vi "Periodic Tasks.vi"(8 "error in":errorcluster) -> ()   [LabVIEW 2023]
doc: "This VI runs in parallel to other tasks. It can contain as many user-defined periodic loops as you need. These can carry out PID or other sorts of timed response."
uses:
  <vilib>/Rock Robotics/WPI/ThirdParty/REV Robotics/REVLib/Typedef/Spark MAX Smart Motion Parameters.ctl
  <vilib>/Rock Robotics/WPI/Utilities/WPI_GetSetVariantRefNum.vi
  <vilib>/Rock Robotics/WPI/RobotDrive/WPI_RobotDriveMecanumDrive_Cartesian.vi
panel:
  in  "Velocity PID Constants RB":T1={"P Gain"=0.0, "I Gain"=0.0, "D Gain"=0.0, "F Gain"=0.0, "I Zone"=0.0, "Min Output"=-1.0, "Max Output"=1.0} {"Max Output" min=-1.0 max=1.0 step=0.01; "Min Output" min=-1.0 max=1.0 step=0.01; "I Zone" step=0.01; "F Gain" step=0.01; "D Gain" step=0.01; "I Gain" step=0.01; "P Gain" min=0.0 step=0.01}
  in  "Smart Motion Parameters RB":T2={"Max Velocity"=2000.0, "Max Acceleration"=1500.0, "Minimum Velocity Output"=0.0, "Allowed Closed Loop Error"=0.0}
  in  "Velocity PID Constants LB":T1={"P Gain"=0.0, "I Gain"=0.0, "D Gain"=0.0, "F Gain"=0.0, "I Zone"=0.0, "Min Output"=-1.0, "Max Output"=1.0} {"Max Output" min=-1.0 max=1.0 step=0.01; "Min Output" min=-1.0 max=1.0 step=0.01; "I Zone" step=0.01; "F Gain" step=0.01; "D Gain" step=0.01; "I Gain" step=0.01; "P Gain" min=0.0 step=0.01}
  in  "Smart Motion Parameters LB":T2={"Max Velocity"=2000.0, "Max Acceleration"=1500.0, "Minimum Velocity Output"=0.0, "Allowed Closed Loop Error"=0.0}
  in  "Velocity PID Constants LF":T1={"P Gain"=0.0, "I Gain"=0.0, "D Gain"=0.0, "F Gain"=0.0, "I Zone"=0.0, "Min Output"=-1.0, "Max Output"=1.0} {"Max Output" min=-1.0 max=1.0 step=0.01; "Min Output" min=-1.0 max=1.0 step=0.01; "I Zone" step=0.01; "F Gain" step=0.01; "D Gain" step=0.01; "I Gain" step=0.01; "P Gain" min=0.0 step=0.01}
  in  "Smart Motion Parameters LF":T2={"Max Velocity"=2000.0, "Max Acceleration"=1500.0, "Minimum Velocity Output"=0.0, "Allowed Closed Loop Error"=0.0}
  in  "Velocity PID Constants RF":T1={"P Gain"=0.0, "I Gain"=0.0, "D Gain"=0.0, "F Gain"=0.0, "I Zone"=0.0, "Min Output"=-1.0, "Max Output"=1.0} {"Max Output" min=-1.0 max=1.0 step=0.01; "Min Output" min=-1.0 max=1.0 step=0.01; "I Zone" step=0.01; "F Gain" step=0.01; "D Gain" step=0.01; "I Gain" step=0.01; "P Gain" min=0.0 step=0.01}
  in  "Smart Motion Parameters RF":T2={"Max Velocity"=2000.0, "Max Acceleration"=1500.0, "Minimum Velocity Output"=0.0, "Allowed Closed Loop Error"=0.0}
  # "Click here to set max"
  # "Click here to set min"
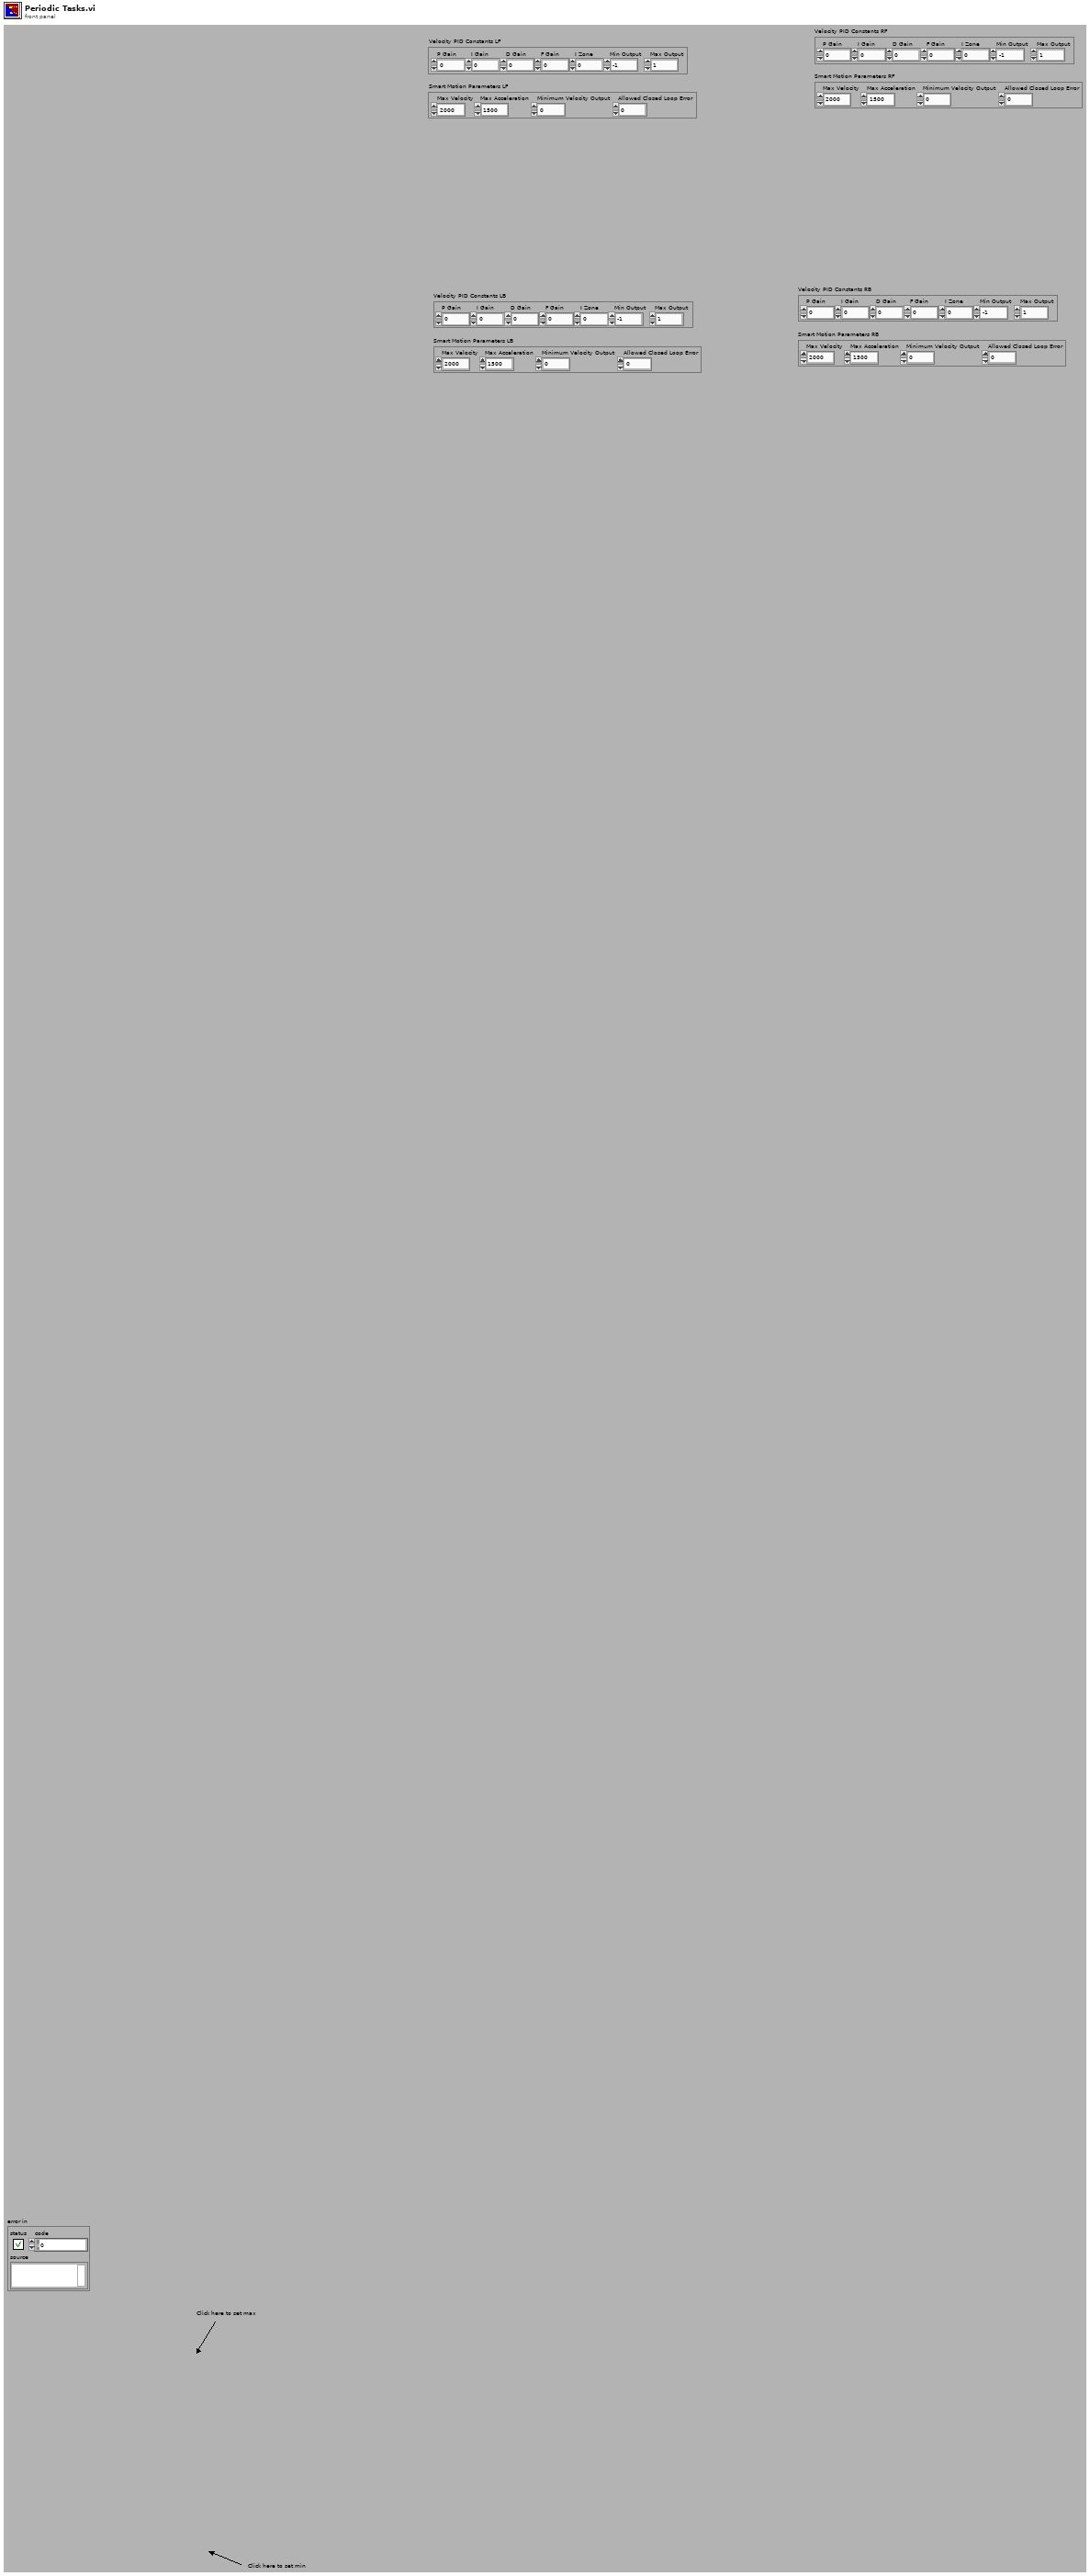
[diagram p1: front panel]
types:
  T1 = cluster{"P Gain":dbl, "I Gain":dbl, "D Gain":dbl, "F Gain":dbl, "I Zone":dbl, "Min Output":dbl, "Max Output":dbl}
  T2 = typedef "Spark MAX Smart Motion Parameters.ctl" = cluster{"Max Velocity":dbl, "Max Acceleration":dbl, "Minimum Velocity Output":dbl, "Allowed Closed Loop Error":dbl}
  T3 = typedef "WPI_JoystickDevRef.ctl" = cluster{"Device":T4}
  T4 = typedef "WPI_JoystickDeviceEnum.ctl" = enum16{"USB 0", "USB 1", "USB 2", "USB 3", "USB 4", "USB 5"}
  T5 = typedef "WPI_RobotDriveDevRef.ctl" = cluster{"DevStatus":errorcluster, "Motors[]":T6[], "Square Inputs":bool, "Max Output":dbl}
  T6 = typedef "WPI_MotorControlDeviceRef.ctl" = cluster{"DeviceStatus":errorcluster, "Type":T7, "PWM":cluster{"PWM Channel":T8, "DeadBand":T9}, "CAN":cluster{"Device Number":u8, "SetOutput VI Ref":variant, "GetOutput VI Ref":variant, "Enable VI Ref":variant, "Disable VI Ref":variant, "Data":variant}, "Invert":bool, "DIO PWM":cluster{"PWM \"Enable\" Channel":T8, "DIOChannel":T10, "PWM Rate":dbl}}
  T7 = typedef "WPI_MotorControlType.ctl" = enum16{"PWM", "CAN", "DIO PWM"}
  T8 = typedef "FPGA_DIOPWMChannel.ctl" = enum8{"PWM 0", "PWM 1", "PWM 2", "PWM 3", "PWM 4", "PWM 5", "PWM 6", "PWM 7", "PWM 8", "PWM 9", "PWM MXP 0", "PWM MXP 1", "PWM MXP 2", "PWM MXP 3", "PWM MXP 4", "PWM MXP 5", "PWM MXP 6", "PWM MXP 7", "PWM MXP 8", "PWM MXP 9", "Invalid"}
  T9 = typedef "WPI_PWMDeadband.ctl" = cluster{"Name":string, "maxPositivePwm":i32, "minPositivePwm":i32, "centerPwm":i32, "maxNegativePwm":i32, "minNegativePwm":i32, "angularRange":u16}
  T10 = typedef "FPGA_DIOChannel.ctl" = enum8{"DIO 0", "DIO 1", "DIO 2", "DIO 3", "DIO 4", "DIO 5", "DIO 6", "DIO 7", "DIO 8", "DIO 9", "DIO MXP 0", "DIO MXP 1", "DIO MXP 2", "DIO MXP 3", "DIO MXP 4", "DIO MXP 5", "DIO MXP 6", "DIO MXP 7", "DIO MXP 8", "DIO MXP 9", "DIO MXP 10", "DIO MXP 11", "DIO MXP 12", "DIO MXP 13", "DIO MXP 14", "DIO MXP 15", "SPI Port CS1", "SPI Port CS2", "SPI Port CS3", "SPI Port MISO", "SPI Port MOSI", "Invalid"}
  T11 = typedef "WPI_DigitalInputDevRef.ctl" = cluster{"DevStatus":errorcluster, "DIO Channel":T10}
  T12 = cluster{"JoystickDevRef":T3, "RobotDriveDevRef":T5}
  T13 = cluster{"P Gain":bool, "I Gain":bool, "D Gain":bool, "F Gain":bool, "I Zone":bool, "Min Output":bool, "Max Output":bool}
  T14 = cluster{"Max Velocity":bool, "Max Acceleration":bool, "Minimum Velocity Output":bool, "Allowed Closed Loop Error":bool}
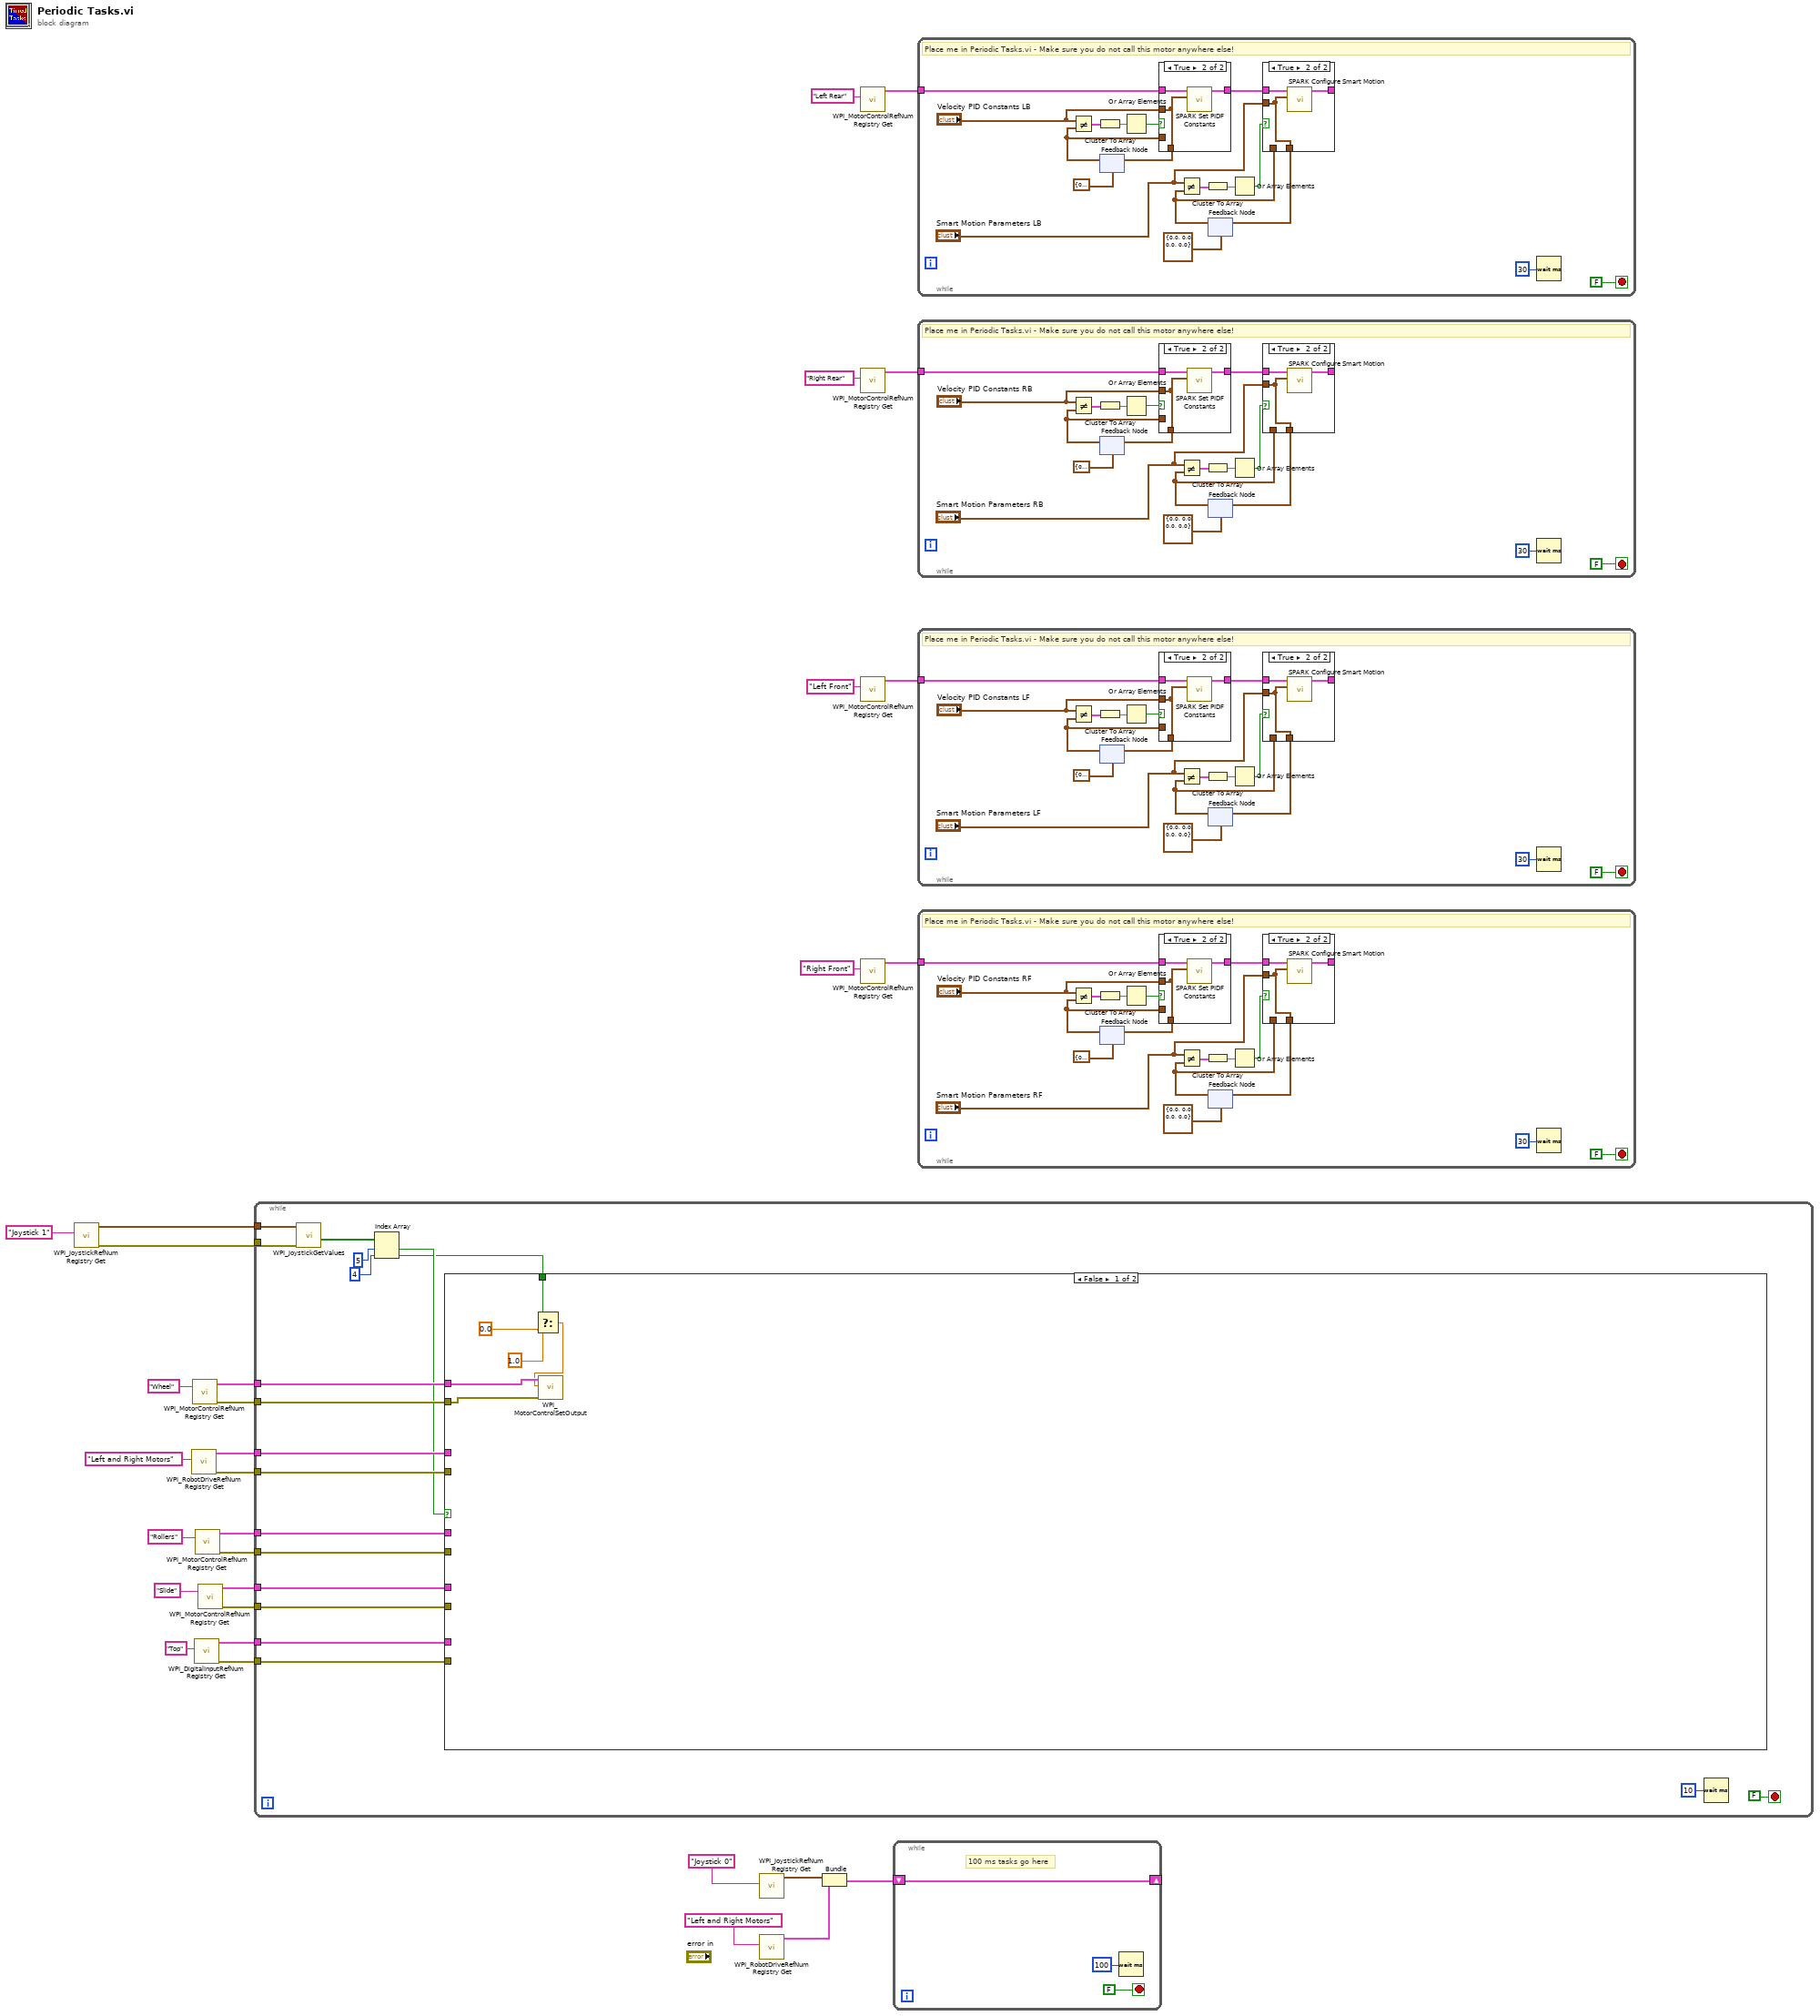
[diagram p0: block diagram]
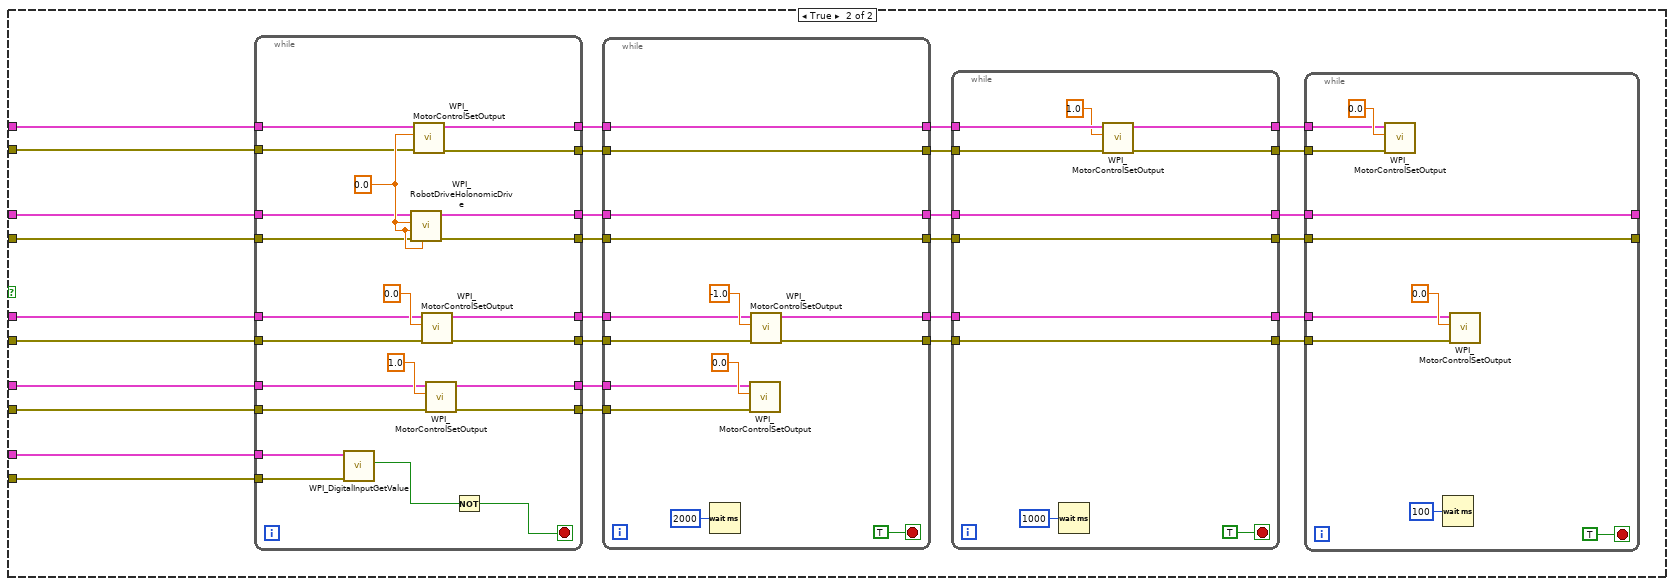
[diagram p10: hidden frame]
diagram:
  n1 = call <vilib>:"WPI_JoystickRefNum Registry Get.vi"("refnum name"="Joystick 1") -> ("error out"=w2:errorcluster, "JoystickDevRef"=w1:T3)  [unwired: 1 in, 8 out]
  n2 = call <vilib>:"WPI_RobotDriveRefNum Registry Get.vi"("refnum name"="Left and Right Motors") -> ("error out"=w5:errorcluster, "RobotDriveDevRef"=w4:T5)  [unwired: 1 in, 8 out]
  n3 = call <vilib>:"WPI_MotorControlRefNum Registry Get.vi"("refnum name"="Wheel") -> ("error out"=w13:errorcluster, "MotorControlDevRef"=w12:T6)  [unwired: 9 in]
  n4 = call <vilib>:"WPI_DigitalInputRefNum Registry Get.vi"("refnum name"="Top") -> ("error out"=w11:errorcluster, "DigitalInputDevRef"=w10:T11)  [unwired: 9 in]
  n5 = call <vilib>:"WPI_MotorControlRefNum Registry Get.vi"("refnum name"="Rollers") -> ("error out"=w7:errorcluster, "MotorControlDevRef"=w6:T6)  [unwired: 9 in]
  n6 = call <vilib>:"WPI_MotorControlRefNum Registry Get.vi"("refnum name"="Slide") -> ("error out"=w9:errorcluster, "MotorControlDevRef"=w8:T6)  [unwired: 9 in]
  n7 = while {
    tunnel: w13 -> [w48]
    tunnel: w12 -> [w47]
    tunnel: w11 -> [w46]
    tunnel: w10 -> [w45]
    tunnel: w9 -> [w44]
    tunnel: w8 -> [w43]
    tunnel: w7 -> [w42]
    tunnel: w6 -> [w41]
    tunnel: w5 -> [w40]
    tunnel: w4 -> [w39]
    tunnel: w2 -> [w37]
    tunnel: w1 -> [w36]
    stop <- FALSE stop-if-true
    n8 = call <vilib>:"WPI_JoystickGetValues.vi"("error in (no error)"=w37, "JoystickDevRef"=w36) -> ("Buttons"=w38:bool[])  [unwired: 5 in, 4 out]
    n9 = Index Array(array=w38, index #1=5 ("index"), index #2=4 ("index")) -> (element #1=w34:bool, element #2=w32:bool)
    n10 = case shown="False" w34 {
      tunnel: w48 -> [w55 w66]
      tunnel: w47 -> [w56 w65]
      tunnel: w46 -> [_ w64]
      tunnel: w45 -> [_ w63]
      tunnel: w44 -> [_ w62]
      tunnel: w43 -> [_ w61]
      tunnel: w42 -> [_ w60]
      tunnel: w41 -> [_ w59]
      tunnel: w40 -> [_ w58]
      tunnel: w39 -> [_ w57]
      tunnel: w32 -> [w51 _]
      frame False {
        n11 = Select(t=1.0 ("Output"), s=w51, f=0.0) -> (s? t:f=w52:dbl)
        n12 = call <vilib>:"WPI_MotorControlSetOutput.vi"("error in (no error)"=w55, "Output"=w52, "MotorControlDevRef"=w56) -> ()  [unwired: 6 in, 3 out]
      }
      frame True {
        n13 = while {
          tunnel: [w129] -> w67
          tunnel: [w128] -> w68
          tunnel: [w126] -> w69
          tunnel: [w125] -> w70
          tunnel: [w122] -> w71
          tunnel: [w121] -> w72
          tunnel: [w119] -> w77
          tunnel: [w118] -> w78
          tunnel: w66 -> [w117]
          tunnel: w65 -> [w116]
          tunnel: w64 -> [w115]
          tunnel: w63 -> [w114]
          tunnel: w62 -> [w113]
          tunnel: w61 -> [w112]
          tunnel: w60 -> [w111]
          tunnel: w59 -> [w110]
          tunnel: w58 -> [w109]
          tunnel: w57 -> [w108]
          stop <- w123 stop-if-true
          w120 = 0.0 ("X")
          n14 = call <vilib>:"WPI_DigitalInputGetValue.vi"("error in (no error)"=w115, "DigitalInputDevRef"=w114) -> ("Value"=w124:bool)  [unwired: 7 in, 2 out]
          n15 = call-poly <vilib>:"WPI_RobotDriveHolonomicDrive.vi"("Rotation"=w120, "error in (no error)"=w109, "Y"=w120, "X"=w120, "RobotDriveDevRef"=w108) -> ("error out"=w122:errorcluster, "RobotDriveDevRef"=w121:T5)  [unwired: 4 in, 1 out]
          n16 = call <vilib>:"WPI_MotorControlSetOutput.vi"("error in (no error)"=w117, "Output"=w120, "MotorControlDevRef"=w116) -> ("error out"=w118:errorcluster, "MotorControlDevRef"=w119:T6)  [unwired: 6 in, 1 out]
          n17 = call <vilib>:"WPI_MotorControlSetOutput.vi"("error in (no error)"=w111, "Output"=0.0, "MotorControlDevRef"=w110) -> ("error out"=w129:errorcluster, "MotorControlDevRef"=w128:T6)  [unwired: 6 in, 1 out]
          n18 = call <vilib>:"WPI_MotorControlSetOutput.vi"("error in (no error)"=w113, "Output"=1.0, "MotorControlDevRef"=w112) -> ("error out"=w125:errorcluster, "MotorControlDevRef"=w126:T6)  [unwired: 6 in, 1 out]
          n19 = Not(x=w124) -> (.not. x?=w123:bool)
        }
        n20 = while {
          tunnel: w67 -> [w143]
          tunnel: w68 -> [w142]
          tunnel: w69 -> [w140]
          tunnel: w70 -> [w139]
          tunnel: [w136] -> w74
          tunnel: w71 -> [w136]
          tunnel: [w135] -> w73
          tunnel: w72 -> [w135]
          tunnel: [w134] -> w75
          tunnel: [w133] -> w76
          tunnel: w77 -> [w132]
          tunnel: w78 -> [w131]
          tunnel: [w132] -> w79
          tunnel: [w131] -> w80
          stop <- TRUE stop-if-true
          n21 = Wait (ms)(milliseconds to wait=u32 2000) -> ()  [unwired: 1 out]
          n22 = call <vilib>:"WPI_MotorControlSetOutput.vi"("error in (no error)"=w139, "Output"=0.0, "MotorControlDevRef"=w140) -> ()  [unwired: 6 in, 3 out]
          n23 = call <vilib>:"WPI_MotorControlSetOutput.vi"("error in (no error)"=w143, "Output"=-1.0, "MotorControlDevRef"=w142) -> ("error out"=w133:errorcluster, "MotorControlDevRef"=w134:T6)  [unwired: 6 in, 1 out]
        }
        n24 = while {
          tunnel: w76 -> [w99]
          tunnel: w75 -> [w100]
          tunnel: [w105] -> w82
          tunnel: w74 -> [w105]
          tunnel: [w104] -> w81
          tunnel: w73 -> [w104]
          tunnel: w79 -> [w103]
          tunnel: w80 -> [w102]
          tunnel: [w100] -> w83
          tunnel: [w99] -> w84
          tunnel: [w98] -> w85
          tunnel: [w97] -> w86
          stop <- TRUE stop-if-true
          n25 = Wait (ms)(milliseconds to wait=u32 1000) -> ()  [unwired: 1 out]
          n26 = call <vilib>:"WPI_MotorControlSetOutput.vi"("error in (no error)"=w102, "Output"=1.0, "MotorControlDevRef"=w103) -> ("error out"=w97:errorcluster, "MotorControlDevRef"=w98:T6)  [unwired: 6 in, 1 out]
        }
        n27 = while {
          tunnel: w81 -> [w94]
          tunnel: [w94] -> _
          tunnel: [w93] -> _
          tunnel: w82 -> [w93]
          tunnel: w83 -> [w92]
          tunnel: w84 -> [w91]
          tunnel: w85 -> [w90]
          tunnel: w86 -> [w89]
          stop <- TRUE stop-if-true
          n28 = call <vilib>:"WPI_MotorControlSetOutput.vi"("error in (no error)"=w89, "Output"=0.0, "MotorControlDevRef"=w90) -> ()  [unwired: 6 in, 3 out]
          n29 = Wait (ms)(milliseconds to wait=u32 100) -> ()  [unwired: 1 out]
          n30 = call <vilib>:"WPI_MotorControlSetOutput.vi"("error in (no error)"=w91, "Output"=0.0, "MotorControlDevRef"=w92) -> ()  [unwired: 6 in, 3 out]
        }
      }
    }
    n31 = Wait (ms)(milliseconds to wait=u32 10) -> ()  [unwired: 1 out]
  }
  n32 = call <vilib>:"WPI_JoystickRefNum Registry Get.vi"("refnum name"="Joystick 0") -> ("JoystickDevRef"=w29:T3)  [unwired: 1 in, 9 out]
  n33 = call <vilib>:"WPI_RobotDriveRefNum Registry Get.vi"("refnum name"="Left and Right Motors") -> ("RobotDriveDevRef"=w28:T5)  [unwired: 1 in, 9 out]
  n34 = Bundle("JoystickDevRef"=w29, "RobotDriveDevRef"=w28) -> (w27:T12)  [unwired: 1 out]
  n35 = call <vilib>:"WPI_MotorControlRefNum Registry Get.vi"("refnum name"="Left Rear") -> ("MotorControlDevRef"=w22:T6)  [unwired: 9 in, 1 out]
  n36 = call <vilib>:"WPI_MotorControlRefNum Registry Get.vi"("refnum name"="Right Rear") -> ("MotorControlDevRef"=w19:T6)  [unwired: 9 in, 1 out]
  n37 = call <vilib>:"WPI_MotorControlRefNum Registry Get.vi"("refnum name"="Left Front") -> ("MotorControlDevRef"=w23:T6)  [unwired: 9 in, 1 out]
  n38 = call <vilib>:"WPI_MotorControlRefNum Registry Get.vi"("refnum name"="Right Front") -> ("MotorControlDevRef"=w26:T6)  [unwired: 9 in, 1 out]
  n39 = while {
    shift-right: [w145] -> _
    shift-left: w27 -> [w145]
    stop <- FALSE stop-if-true
    # "100 ms tasks go here"
    n40 = Wait (ms)(milliseconds to wait=u32 100) -> ()  [unwired: 1 out]
  }
  n41 = while {
    tunnel: w22 -> [w156]
    stop <- FALSE stop-if-true
    # "Place me in Periodic Tasks.vi - Make sure you do not call this motor anywhere else!"
    n42 = feedback #1(T1 {"P Gain"=0.0, "I Gain"=0.0, "D Gain"=0.0, "F Gain"=0.0, "I Zone"=0.0, "Min Output"=0.0, "Max Output"=0.0} ("PID Constants")) -> (w165:T1)
    n43 = Not Equal?(x="Velocity PID Constants LB", y=w165) -> (x != y?=w159:T13)
    n44 = Cluster To Array(cluster=w159) -> (array=w160:bool[])
    n45 = Or Array Elements(Boolean array=w160) -> (logical OR=w162:bool)
    n46 = case shown="True" w162 {
      tunnel: w156 -> [w171 w175]
      tunnel: "Velocity PID Constants LB" -> [_ w173]
      tunnel: [w172 w173] -> w164
      tunnel: w165 -> [w172 _]
      tunnel: [w171 w174] -> w155
      frame False {
      }
      frame True {
        n47 = call <vilib>:"SPARK Set PIDF Constants.vi"("PID Constants"=w173, "MotorControlDeviceRef"=w175) -> ("MotorControlDeviceRef"=w174:T6)  [unwired: 8 in, 1 out]
      }
    }
    n48 = feedback-in #1(w164) -> ()
    n49 = feedback #2(T2 {"Max Velocity"=0.0, "Max Acceleration"=0.0, "Minimum Velocity Output"=0.0, "Allowed Closed Loop Error"=0.0} ("Smart Motion Parameters")) -> (w148:T2)
    n50 = Not Equal?(x="Smart Motion Parameters LB", y=w148) -> (x != y?=w153:T14)
    n51 = Cluster To Array(cluster=w153) -> (array=w154:bool[])
    n52 = Or Array Elements(Boolean array=w154) -> (logical OR=w152:bool)
    n53 = case shown="True" w152 {
      tunnel: w155 -> [w167 w170]
      tunnel: "Smart Motion Parameters LB" -> [_ w168]
      tunnel: [w167 w169] -> _
      tunnel: [w166 w168] -> w149
      tunnel: w148 -> [w166 _]
      frame False {
      }
      frame True {
        n54 = call <vilib>:"SPARK Configure Smart Motion.vi"("Smart Motion Parameters"=w168, "MotorControlDeviceRef"=w170) -> ("MotorControlDeviceRef"=w169:T6)  [unwired: 8 in, 1 out]
      }
    }
    n55 = feedback-in #2(w149) -> ()
    n56 = Wait (ms)(milliseconds to wait=u32 30) -> ()  [unwired: 1 out]
  }
  n57 = while {
    tunnel: w19 -> [w184]
    stop <- FALSE stop-if-true
    # "Place me in Periodic Tasks.vi - Make sure you do not call this motor anywhere else!"
    n58 = feedback #3(T1 {"P Gain"=0.0, "I Gain"=0.0, "D Gain"=0.0, "F Gain"=0.0, "I Zone"=0.0, "Min Output"=0.0, "Max Output"=0.0} ("PID Constants")) -> (w193:T1)
    n59 = Not Equal?(x="Velocity PID Constants RB", y=w193) -> (x != y?=w187:T13)
    n60 = Cluster To Array(cluster=w187) -> (array=w188:bool[])
    n61 = Or Array Elements(Boolean array=w188) -> (logical OR=w190:bool)
    n62 = case shown="True" w190 {
      tunnel: w184 -> [w199 w203]
      tunnel: "Velocity PID Constants RB" -> [_ w201]
      tunnel: [w200 w201] -> w192
      tunnel: w193 -> [w200 _]
      tunnel: [w199 w202] -> w183
      frame False {
      }
      frame True {
        n63 = call <vilib>:"SPARK Set PIDF Constants.vi"("PID Constants"=w201, "MotorControlDeviceRef"=w203) -> ("MotorControlDeviceRef"=w202:T6)  [unwired: 8 in, 1 out]
      }
    }
    n64 = feedback-in #3(w192) -> ()
    n65 = feedback #4(T2 {"Max Velocity"=0.0, "Max Acceleration"=0.0, "Minimum Velocity Output"=0.0, "Allowed Closed Loop Error"=0.0} ("Smart Motion Parameters")) -> (w176:T2)
    n66 = Not Equal?(x="Smart Motion Parameters RB", y=w176) -> (x != y?=w181:T14)
    n67 = Cluster To Array(cluster=w181) -> (array=w182:bool[])
    n68 = Or Array Elements(Boolean array=w182) -> (logical OR=w180:bool)
    n69 = case shown="True" w180 {
      tunnel: w183 -> [w195 w198]
      tunnel: "Smart Motion Parameters RB" -> [_ w196]
      tunnel: [w195 w197] -> _
      tunnel: [w194 w196] -> w177
      tunnel: w176 -> [w194 _]
      frame False {
      }
      frame True {
        n70 = call <vilib>:"SPARK Configure Smart Motion.vi"("Smart Motion Parameters"=w196, "MotorControlDeviceRef"=w198) -> ("MotorControlDeviceRef"=w197:T6)  [unwired: 8 in, 1 out]
      }
    }
    n71 = feedback-in #4(w177) -> ()
    n72 = Wait (ms)(milliseconds to wait=u32 30) -> ()  [unwired: 1 out]
  }
  n73 = while {
    tunnel: w23 -> [w212]
    stop <- FALSE stop-if-true
    # "Place me in Periodic Tasks.vi - Make sure you do not call this motor anywhere else!"
    n74 = feedback #5(T1 {"P Gain"=0.0, "I Gain"=0.0, "D Gain"=0.0, "F Gain"=0.0, "I Zone"=0.0, "Min Output"=0.0, "Max Output"=0.0} ("PID Constants")) -> (w221:T1)
    n75 = Not Equal?(x="Velocity PID Constants LF", y=w221) -> (x != y?=w215:T13)
    n76 = Cluster To Array(cluster=w215) -> (array=w216:bool[])
    n77 = Or Array Elements(Boolean array=w216) -> (logical OR=w218:bool)
    n78 = case shown="True" w218 {
      tunnel: w212 -> [w227 w231]
      tunnel: "Velocity PID Constants LF" -> [_ w229]
      tunnel: [w228 w229] -> w220
      tunnel: w221 -> [w228 _]
      tunnel: [w227 w230] -> w211
      frame False {
      }
      frame True {
        n79 = call <vilib>:"SPARK Set PIDF Constants.vi"("PID Constants"=w229, "MotorControlDeviceRef"=w231) -> ("MotorControlDeviceRef"=w230:T6)  [unwired: 8 in, 1 out]
      }
    }
    n80 = feedback-in #5(w220) -> ()
    n81 = feedback #6(T2 {"Max Velocity"=0.0, "Max Acceleration"=0.0, "Minimum Velocity Output"=0.0, "Allowed Closed Loop Error"=0.0} ("Smart Motion Parameters")) -> (w204:T2)
    n82 = Not Equal?(x="Smart Motion Parameters LF", y=w204) -> (x != y?=w209:T14)
    n83 = Cluster To Array(cluster=w209) -> (array=w210:bool[])
    n84 = Or Array Elements(Boolean array=w210) -> (logical OR=w208:bool)
    n85 = case shown="True" w208 {
      tunnel: w211 -> [w223 w226]
      tunnel: "Smart Motion Parameters LF" -> [_ w224]
      tunnel: [w223 w225] -> _
      tunnel: [w222 w224] -> w205
      tunnel: w204 -> [w222 _]
      frame False {
      }
      frame True {
        n86 = call <vilib>:"SPARK Configure Smart Motion.vi"("Smart Motion Parameters"=w224, "MotorControlDeviceRef"=w226) -> ("MotorControlDeviceRef"=w225:T6)  [unwired: 8 in, 1 out]
      }
    }
    n87 = feedback-in #6(w205) -> ()
    n88 = Wait (ms)(milliseconds to wait=u32 30) -> ()  [unwired: 1 out]
  }
  n89 = while {
    tunnel: w26 -> [w240]
    stop <- FALSE stop-if-true
    # "Place me in Periodic Tasks.vi - Make sure you do not call this motor anywhere else!"
    n90 = feedback #7(T1 {"P Gain"=0.0, "I Gain"=0.0, "D Gain"=0.0, "F Gain"=0.0, "I Zone"=0.0, "Min Output"=0.0, "Max Output"=0.0} ("PID Constants")) -> (w249:T1)
    n91 = Not Equal?(x="Velocity PID Constants RF", y=w249) -> (x != y?=w243:T13)
    n92 = Cluster To Array(cluster=w243) -> (array=w244:bool[])
    n93 = Or Array Elements(Boolean array=w244) -> (logical OR=w246:bool)
    n94 = case shown="True" w246 {
      tunnel: w240 -> [w255 w259]
      tunnel: "Velocity PID Constants RF" -> [_ w257]
      tunnel: [w256 w257] -> w248
      tunnel: w249 -> [w256 _]
      tunnel: [w255 w258] -> w239
      frame False {
      }
      frame True {
        n95 = call <vilib>:"SPARK Set PIDF Constants.vi"("PID Constants"=w257, "MotorControlDeviceRef"=w259) -> ("MotorControlDeviceRef"=w258:T6)  [unwired: 8 in, 1 out]
      }
    }
    n96 = feedback-in #7(w248) -> ()
    n97 = feedback #8(T2 {"Max Velocity"=0.0, "Max Acceleration"=0.0, "Minimum Velocity Output"=0.0, "Allowed Closed Loop Error"=0.0} ("Smart Motion Parameters")) -> (w232:T2)
    n98 = Not Equal?(x="Smart Motion Parameters RF", y=w232) -> (x != y?=w237:T14)
    n99 = Cluster To Array(cluster=w237) -> (array=w238:bool[])
    n100 = Or Array Elements(Boolean array=w238) -> (logical OR=w236:bool)
    n101 = case shown="True" w236 {
      tunnel: w239 -> [w251 w254]
      tunnel: "Smart Motion Parameters RF" -> [_ w252]
      tunnel: [w251 w253] -> _
      tunnel: [w250 w252] -> w233
      tunnel: w232 -> [w250 _]
      frame False {
      }
      frame True {
        n102 = call <vilib>:"SPARK Configure Smart Motion.vi"("Smart Motion Parameters"=w252, "MotorControlDeviceRef"=w254) -> ("MotorControlDeviceRef"=w253:T6)  [unwired: 8 in, 1 out]
      }
    }
    n103 = feedback-in #8(w233) -> ()
    n104 = Wait (ms)(milliseconds to wait=u32 30) -> ()  [unwired: 1 out]
  }
